vi "calibrateArmEncoder.vi"   [LabVIEW 2015]
uses:
  Robot Global Data.vi
types:
  T1 = typedef "WPI_MotorControlDeviceRef.ctl" = cluster{"DeviceStatus":errorcluster, "Type":T2, "PWM":cluster{"PWM Channel":T3, "DeadBand":T4}, "CAN":cluster{"Device Number":u8, "Control Mode":T5, "Semaphore":T6, "Max Vout":dbl, "TalonSRX Control Mode":T7}, "Invert":bool}
  T2 = typedef "WPI_MotorControlType.ctl" = enum16{"PWM", "CAN", "CANTalonSRX"}
  T3 = typedef "FPGA_DIOPWMChannel.ctl" = enum8{"PWM 0", "PWM 1", "PWM 2", "PWM 3", "PWM 4", "PWM 5", "PWM 6", "PWM 7", "PWM 8", "PWM 9", "PWM MXP 0", "PWM MXP 1", "PWM MXP 2", "PWM MXP 3", "PWM MXP 4", "PWM MXP 5", "PWM MXP 6", "PWM MXP 7", "PWM MXP 8", "PWM MXP 9", "Invalid"}
  T4 = typedef "WPI_PWMDeadband.ctl" = cluster{"Name":string, "maxPositivePwm":i32, "minPositivePwm":i32, "centerPwm":i32, "maxNegativePwm":i32, "minNegativePwm":i32, "angularRange":u16}
  T5 = typedef "WPI_CANJaguar_ControlMode.ctl" = enum8{"Percent VBus", "Current", "Speed", "Position", "Voltage"}
  T6 = typedef "Semaphore RefNum" = refnum<k1>
  T7 = typedef "WPI_CANTalonSRX_APIControlMode.ctl" = enum8{"Percent VBus", "Speed", "Position", "Slave", "Unchanged / Invalid", "Voltage Compensation", "Current", "Motion Profile"}
  T8 = typedef "WPI_SwitchDevRef.ctl" = cluster{"DevStatus":errorcluster, "DIO Channel":T9, "CntIndex":T10, "Normally Closed":bool}
  T9 = typedef "FPGA_DIOChannel.ctl" = enum8{"DIO 0", "DIO 1", "DIO 2", "DIO 3", "DIO 4", "DIO 5", "DIO 6", "DIO 7", "DIO 8", "DIO 9", "DIO MXP 0", "DIO MXP 1", "DIO MXP 2", "DIO MXP 3", "DIO MXP 4", "DIO MXP 5", "DIO MXP 6", "DIO MXP 7", "DIO MXP 8", "DIO MXP 9", "DIO MXP 10", "DIO MXP 11", "DIO MXP 12", "DIO MXP 13", "DIO MXP 14", "DIO MXP 15", "Invalid"}
  T10 = typedef "FPGA_CounterCtrSystemIndex.ctl" = enum8{"Ctr 0", "Ctr 1", "Ctr 2", "Ctr 3", "Ctr 4", "Ctr 5", "Ctr 6", "Ctr 7", "Invalid"}
  T11 = typedef "WPI_PotentiometerDevRef.ctl" = cluster{"DevStatus":errorcluster, "Analog Channel":T12, "Invert Output":bool}
  T12 = typedef "FPGA_AIChannel.ctl" = enum8{"AI 0", "AI 1", "AI 2", "AI 3", "AI MXP 0", "AI MXP 1", "AI MXP 2", "AI MXP 3", "Invalid"}
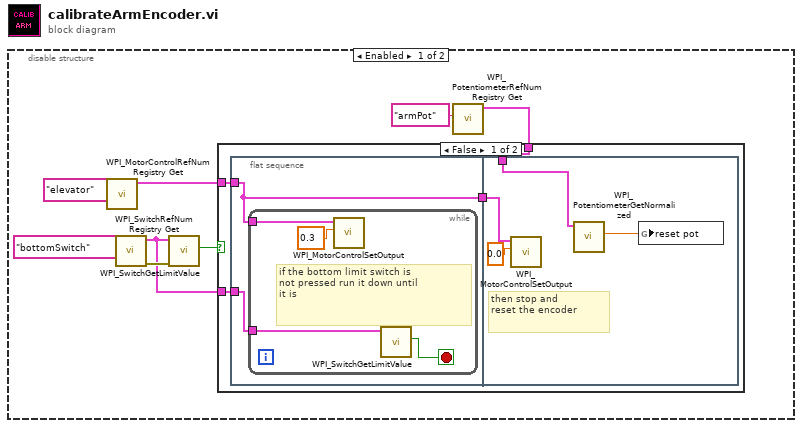
[diagram p0: block diagram]
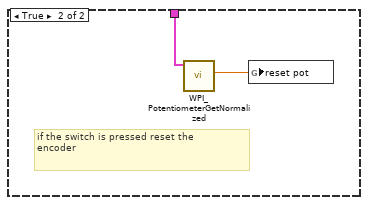
[diagram p2: hidden frame]
diagram:
  n1 = disable-structure shown="Enabled" {
    frame Enabled {
      n2 = call <vilib>:"WPI_MotorControlRefNum Registry Get.vi"("refnum name"="elevator") -> ("MotorControlDevRef"=w7:T1)  [unwired: 9 in, 1 out]
      n3 = call <vilib>:"WPI_SwitchRefNum Registry Get.vi"("refnum name"="bottomSwitch") -> ("error out"=w4:errorcluster, "SwitchDevRef"=w2:T8)  [unwired: 9 in]
      n4 = call <vilib>:"WPI_SwitchGetLimitValue.vi"("error in (no error)"=w4, "SwitchDevRef"=w2) -> ("Switch Pressed"=w5:bool)  [unwired: 7 in, 2 out]
      n5 = call <vilib>:"WPI_PotentiometerRefNum Registry Get.vi"("refnum name"="armPot") -> ("PotDevRef"=w1:T11)  [unwired: 9 in, 1 out]
      n6 = case shown="False" w5 {
        tunnel: w7 -> [w12 _]
        tunnel: w2 -> [w10 _]
        tunnel: w1 -> [w9 w23]
        frame False {
          n7 = flat-sequence {
            tunnel: w12 -> [w13]
            tunnel: [w13] -> w11
            tunnel: w10 -> [w14]
            tunnel: w11 -> [w22]
            tunnel: w9 -> [w20]
            frame #0 {
              n8 = while {
                tunnel: w13 -> [w17]
                tunnel: w14 -> [w15]
                stop <- w16 stop-if-true
                # "if the bottom limit switch is \nnot pressed run it down until\nit is"
                n9 = call <vilib>:"WPI_MotorControlSetOutput.vi"("Output"=0.3, "MotorControlDevRef"=w17) -> ()  [unwired: 7 in, 3 out]
                n10 = call <vilib>:"WPI_SwitchGetLimitValue.vi"("SwitchDevRef"=w15) -> ("Switch Pressed"=w16:bool)  [unwired: 8 in, 2 out]
              }
            }
            frame #1 {
              # "then stop and\nreset the encoder"
              n11 = call <vilib>:"WPI_MotorControlSetOutput.vi"("Output"=0.0, "MotorControlDevRef"=w22) -> ()  [unwired: 7 in, 3 out]
              n12 = call <vilib>:"WPI_PotentiometerGetNormalized.vi"("PotDevRef"=w20) -> ("Normalized Value"=w19:dbl)  [unwired: 8 in, 2 out]
              n13 = global write "Robot Global Data.vi" "reset pot"(w19) -> ()
            }
          }
        }
        frame True {
          # "if the switch is pressed reset the\nencoder"
          n14 = call <vilib>:"WPI_PotentiometerGetNormalized.vi"("PotDevRef"=w23) -> ("Normalized Value"=w24:dbl)  [unwired: 8 in, 2 out]
          n15 = global write "Robot Global Data.vi" "reset pot"(w24) -> ()
        }
      }
    }
    frame Disabled {
    }
  }
